vi "MSScript_Error_(6008)UnknownCmd.vi"(0 "error in (no error)":errorcluster, 1 "ErrBoolean":bool) -> (2 "error out":errorcluster)   [LabVIEW 2018, in "MSScript.lvclass"]
uses:
  MSScript.lvclass
  <vilib>/Utility/error.llb/Error Cluster From Error Code.vi
  <vilib>/ErrorRing/Error Ring.xnode
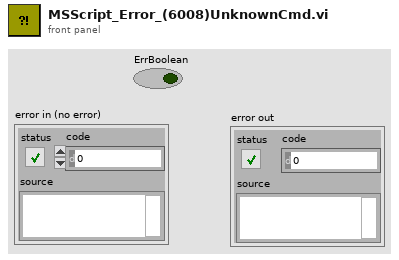
[diagram p1: front panel]
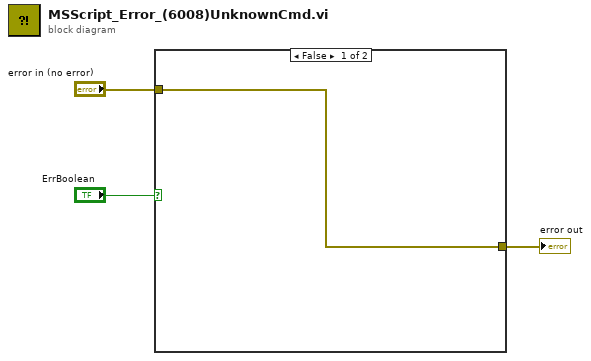
[diagram p0: block diagram]
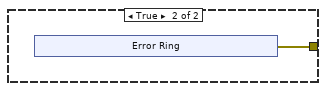
[diagram p2: hidden frame]
diagram:
  n1 = case shown="False" "ErrBoolean" {
    tunnel: "error in (no error)" -> [w4 _]
    tunnel: [w4 w5] -> w1
    frame False {
    }
    frame True {
      n2 = xnode "Error Ring"() -> ("error out"=w5:errorcluster)
    }
  }
  "error out" <- w1
